vi "Swerve Wheel Position.vi"() -> ()   [LabVIEW 2016]
uses:
  <vilib>/Rock Robotics/Network Tables/NT Read Number.vi
  <vilib>/Rock Robotics/Network Tables/NT Write Number.vi
panel:
  in  "Deadband":dbl
  in  "Input Array":dbl[](array[numeric])
  out "Drive Output":dbl
  in  "Wheel":T1(ring)
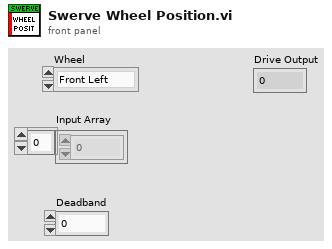
[diagram p1: front panel]
types:
  T1 = enum16{"Front Left", "Front Right", "Back Left", "Back Right"}
  T2 = enum16{"Z", "Y", "X", "Rot. Point X", "Rot. Point Y", "Width/2", "Max", "Length/2"}
  T3 = enum16{"Z Axis", "Y", "X", "Rot. Point X", "Rot. Point Y", "Width/2", "Max", "Length/2"}
  T4 = typedef "WPI_MotorControlDeviceRef.ctl" = cluster{"DeviceStatus":errorcluster, "Type":T5, "PWM":cluster{"PWM Channel":T6, "DeadBand":T7}, "CAN":cluster{"Device Number":u8, "SetOutput VI Ref":variant, "GetOutput VI Ref":variant, "Enable VI Ref":variant, "Disable VI Ref":variant, "Data":variant}, "Invert":bool}
  T5 = typedef "WPI_MotorControlType.ctl" = enum16{"PWM", "CAN"}
  T6 = typedef "FPGA_DIOPWMChannel.ctl" = enum8{"PWM 0", "PWM 1", "PWM 2", "PWM 3", "PWM 4", "PWM 5", "PWM 6", "PWM 7", "PWM 8", "PWM 9", "PWM MXP 0", "PWM MXP 1", "PWM MXP 2", "PWM MXP 3", "PWM MXP 4", "PWM MXP 5", "PWM MXP 6", "PWM MXP 7", "PWM MXP 8", "PWM MXP 9", "Invalid"}
  T7 = typedef "WPI_PWMDeadband.ctl" = cluster{"Name":string, "maxPositivePwm":i32, "minPositivePwm":i32, "centerPwm":i32, "maxNegativePwm":i32, "minNegativePwm":i32, "angularRange":u16}
  T8 = typedef "WPI_CANTalonSRX_GlobalStatus.ctl" = cluster{"Applied Throttle":dbl, "Module Enabled":bool, "CAN Error":errorcluster, "Closed Loop Error":dbl, "Forward Limit Switch Closed":bool, "Reverse Limit Switch Closed":bool, "Sensor Position":dbl, "Sensor Velocity":dbl, "Current":dbl, "Sticky Fault - Over Temp":bool, "Sticky Fault - Under Voltage":bool, "Sticky Fault - Forward Limit":bool, "Sticky Fault - Reverse Limit":bool, "Sticky Fault - Forward Soft Limit":bool, "Sticky Fault - Reverse Soft Limit":bool, "Brake is Enabled":bool, "Encoder Position":dbl, "Encoder Velocity":dbl, "Encoder Index Count":dbl, "Encoder A Pin State":bool, "Encoder B Pin State":bool, "Encoder Index Pin State":bool, "Analog In":dbl, "Analog In Velocity":dbl, "Temperature (C)":dbl, "Battery Voltage":dbl, "Control 5 Is Supported":bool, "Current Profile Slot Select":dbl, "Pos Div 8":bool, "Vel Div 4":bool, "Pulse Width Position":i32, "Pulse Width Velocity":i32, "Pulse Width Rise To Rise (us)":i32, "Pulse Width Rise To Fall (us)":i32, "Mot Prof Active Is Under Run":bool, "Mot Prof Active Has Under Run":bool, "Mot Prof Active Is Last":bool, "Mot Prof Active Velocity Only":bool, "Mot Prof Active Is Valid":bool, "Mot Prof Buffer Is Full":bool, "Mot Prof Active Profile Slot Select":i32, "Mot Prof NextID":i32, "Mot Prof Count":i32, "Mot Prof Active Velocity":dbl, "Mot Prof Active Position":dbl, "Mot Prof Output Enable":i32, "UsageFrame":u32}
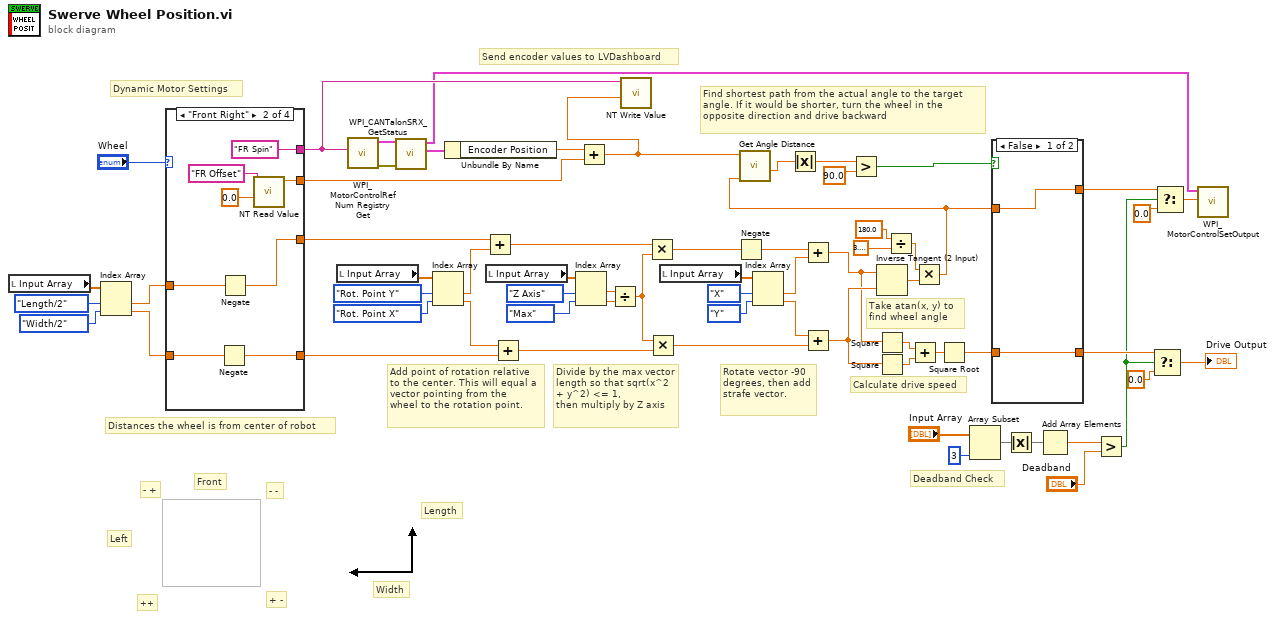
[diagram p0: block diagram]
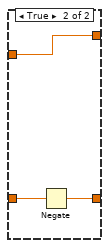
[diagram p2: hidden frame]
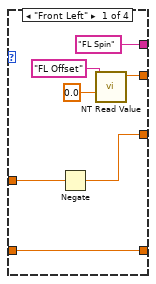
[diagram p3: hidden frame]
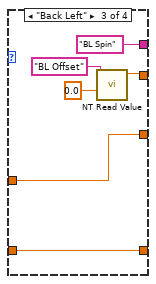
[diagram p4: hidden frame]
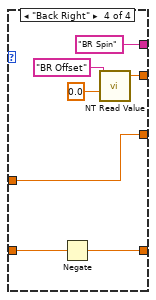
[diagram p5: hidden frame]
diagram:
  # "Take atan(x, y) to find wheel angle"
  # "Calculate drive speed"
  # "- -"
  # "+ -"
  # "++"
  # "- +"
  # "Width"
  # "Length"
  # "Left"
  # "Front"
  # "Distances the wheel is from center of robot"
  # "Dynamic Motor Settings"
  # "Divide by the max vector length so that sqrt(x^2 + y^2) <= 1,\nthen multiply by Z axis"
  # "Add point of rotation relative to the center. This will equal a vector pointing from the\nwheel to the rotation point."
  # "Rotate vector -90 degrees, then add strafe vector."
  # "Deadband Check"
  # "Find shortest path from the actual angle to the target angle. If it would be shorter, turn the wheel in the opposite direction and drive backward"
  # "Send encoder values to LVDashboard"
  n1 = local read "Input Array"() -> (w29:dbl[])
  n2 = Index Array(array=w29, index #1=T2."Length/2", index #2=T2."Width/2") -> (element #1=w25:dbl, element #2=w24:dbl)
  n3 = case shown="\"Front Right\"" "Wheel" {
    tunnel: ["FL Spin" ("refnum name") "FR Spin" ("refnum name") "BL Spin" ("refnum name") "BR Spin" ("refnum name")] -> w61
    tunnel: [w69 w77 w83 w90] -> w2
    tunnel: [w66 w74 w82 w89] -> w27
    tunnel: w25 -> [w68 w76 w82 w89]
    tunnel: [w67 w73 w81 w87] -> w26
    tunnel: w24 -> [w67 w75 w81 w88]
    frame "Front Left" {
      n4 = Negate(x=w68) -> (-x=w66:dbl)
      n5 = call-poly <vilib>:"NT Read Value.vi"("Default Value"=0.0, "Name"="FL Offset") -> ("Numeric"=w69:dbl)  [unwired: 8 in, 1 out]
    }
    frame "Front Right" {
      n6 = Negate(x=w75) -> (-x=w73:dbl)
      n7 = Negate(x=w76) -> (-x=w74:dbl)
      n8 = call-poly <vilib>:"NT Read Value.vi"("Default Value"=0.0, "Name"="FR Offset") -> ("Numeric"=w77:dbl)  [unwired: 8 in, 1 out]
    }
    frame "Back Left" {
      n9 = call-poly <vilib>:"NT Read Value.vi"("Default Value"=0.0, "Name"="BL Offset") -> ("Numeric"=w83:dbl)  [unwired: 8 in, 1 out]
    }
    frame "Back Right" {
      n10 = Negate(x=w88) -> (-x=w87:dbl)
      n11 = call-poly <vilib>:"NT Read Value.vi"("Default Value"=0.0, "Name"="BR Offset") -> ("Numeric"=w90:dbl)  [unwired: 8 in, 1 out]
    }
  }
  n12 = local read "Input Array"() -> (w50:dbl[])
  n13 = call <vilib>:"WPI_MotorControlRefNum Registry Get.vi"("refnum name"=w61) -> ("error out"=w63:errorcluster, "MotorControlDevRef"=w64:T4)  [unwired: 9 in]
  n14 = call <vilib>:"WPI_CANTalonSRX_GetStatus.vi"("error in (no error)"=w63, "CAN Talon SRX Ref"=w64) -> ("Talon SRX Status"=w62:T8, "CAN Talon SRX Ref"=w6:T4)  [unwired: 7 in, 1 out]
  n15 = Index Array(array=w50, index #1=T2."Rot. Point Y", index #2=T2."Rot. Point X") -> (element #1=w47:dbl, element #2=w48:dbl)
  n16 = Unbundle By Name(w62) -> ("Encoder Position"=w60:dbl)
  n17 = Add(x=w27, y=w47) -> (x+y=w31:dbl)
  n18 = local read "Input Array"() -> (w45:dbl[])
  n19 = Add(x=w48, y=w26) -> (x+y=w41:dbl)
  n20 = Index Array(array=w45, index #1=T3."Z Axis", index #2=T2."Max") -> (element #1=w42:dbl, element #2=w43:dbl)
  n21 = Add(x=w60, y=w2) -> (x+y=w1:dbl)
  n22 = Divide(x=w42, y=w43) -> (x/y=w40:dbl)
  n23 = call-poly <vilib>:"NT Write Value.vi"("Numeric"=w1, "Name"=w61) -> ()  [unwired: 9 in, 1 out]
  n24 = Multiply(x=w31, y=w40) -> (x*y=w33:dbl)
  n25 = Multiply(x=w40, y=w41) -> (x*y=w36:dbl)
  n26 = local read "Input Array"() -> (w38:dbl[])
  n27 = Negate(x=w33) -> (-x=w32:dbl)
  n28 = Index Array(array=w38, index #1=T2."X", index #2=T2."Y") -> (element #1=w34:dbl, element #2=w35:dbl)
  n29 = Add(x=w32, y=w34) -> (x+y=w15:dbl)
  n30 = Add(x=w35, y=w36) -> (x+y=w16:dbl)
  n31 = Inverse Tangent (2 Input)(1:w16, 2:w15) -> (0:w23:dbl)
  n32 = Square(x=w15) -> (x^2=w17:dbl)
  n33 = Square(x=w16) -> (x^2=w22:dbl)
  n34 = Divide(x=180.0 ("y"), y=3.141592653589793) -> (x/y=w20:dbl)
  n35 = Add(x=w17, y=w22) -> (x+y=w21:dbl)
  n36 = Multiply(x=w20, y=w23) -> (x*y=w3:dbl)
  n37 = call "Get Angle Distance.vi"("Target"=w3, "Current"=w1) -> ("Distance"=w11:dbl)  [unwired: 9 in]
  n38 = Absolute Value(x=w11) -> (abs(x)=w13:dbl)
  n39 = Greater?(x=w13, y=90.0) -> (0:w12:bool)
  n40 = Square Root(x=w21) -> (sqrt(x)=w9:dbl)
  n41 = Array Subset(array="Input Array", length=3) -> (w57:dbl[])  [unwired: 1 in]
  n42 = case shown="False" w12 {
    tunnel: [w95 w97] -> w10
    tunnel: w9 -> [w95 w98]
    tunnel: [w94 w96] -> w4
    tunnel: w3 -> [w94 w96]
    frame False {
    }
    frame True {
      n43 = Negate(x=w98) -> (-x=w97:dbl)
    }
  }
  n44 = Absolute Value(x=w57) -> (abs(x)=w55:dbl[])
  n45 = Add Array Elements(numeric array=w55) -> (sum=w53:dbl)
  n46 = Greater?(x=w53, y="Deadband") -> (0:w5:bool)
  n47 = Select(t=w10, s=w5, f=0.0) -> (s? t:f=→"Drive Output":dbl)
  n48 = Select(t=w4, s=w5, f=0.0) -> (s? t:f=w8:dbl)
  n49 = call <vilib>:"WPI_MotorControlSetOutput.vi"("Output"=w8, "MotorControlDevRef"=w6) -> ()  [unwired: 7 in, 3 out]
